vi "Acquire DI Data.vi"(6 "Simulate":bool, 7 "IONames[]":string[](array[string]), 8 "error in":errorcluster, 11 "task in":refnum<k21>) -> (0 "error out":errorcluster, 2 "data":bool[](array[boolean]))   [LabVIEW 2017]
uses:
  <vilib>/DAQmx/read.llb/DAQmx Read (Digital 1D Bool NChan 1Samp 1Line).vi
  <vilib>/DAQmx/miscellaneous.llb/DAQmx Fill In Error Info.vi
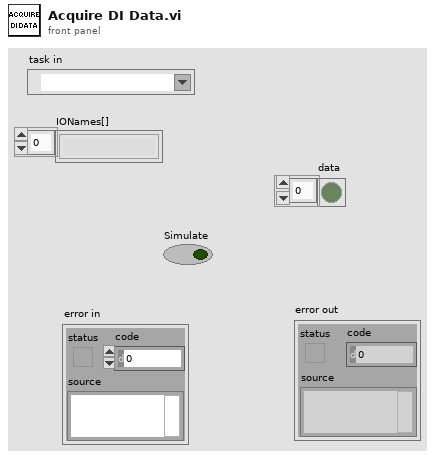
[diagram p1: front panel]
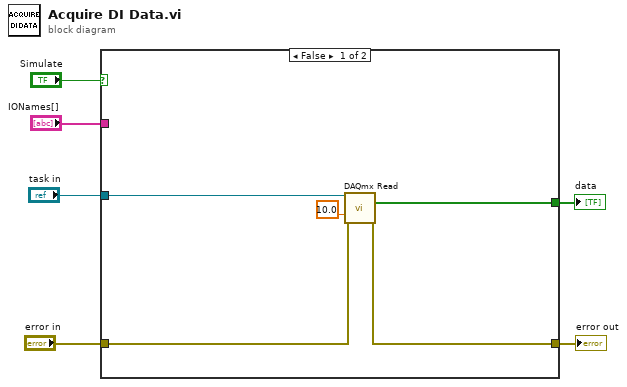
[diagram p0: block diagram]
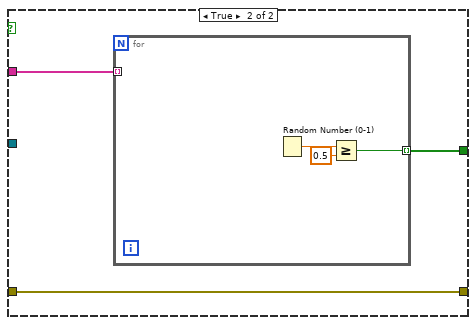
[diagram p2: hidden frame]
diagram:
  n1 = case shown="False" "Simulate" {
    tunnel: "task in" -> [w7 _]
    tunnel: "error in" -> [w9 w13]
    tunnel: [w10 w13] -> w4
    tunnel: "IONames[]" -> [_ w14]
    tunnel: [w8 w12] -> w1
    frame False {
      n2 = call-poly <vilib>:"DAQmx Read.vi"("task/channels in"=w7, "timeout"=10.0, "error in"=w9) -> ("data"=w8:bool[], "error out"=w10:errorcluster)  [unwired: 10 in, 1 out]
    }
    frame True {
      n3 = for {
        tunnel: w14 -> [_] mode=indexing
        tunnel: [w15] -> w12 mode=indexing
        n4 = Random Number (0-1)() -> (number: 0 to 1=w17:dbl)
        n5 = Greater Or Equal?(x=w17, y=0.5) -> (x >= y?=w15:bool)
      }
    }
  }
  "error out" <- w4
  "data" <- w1
